vi "Get Groups Channels and Properties from Tags.vi"(6 "error in":errorcluster, 8 "File Tree":string[](array[string]), 9 "tdms file in":refnum<k34>) -> (0 "error out":errorcluster, 1 "channel names out":string[](array[string]), 2 "group names out":string[](array[string]), 3 "tdms file out":refnum<k34>, 4 "property table":string[][](array[string]))   [LabVIEW 2020, in "NI_TDMS File Viewer.lvlib"]
uses:
  <vilib>/Utility/TDMS File Viewer/NI_TDMS File Viewer.lvlib
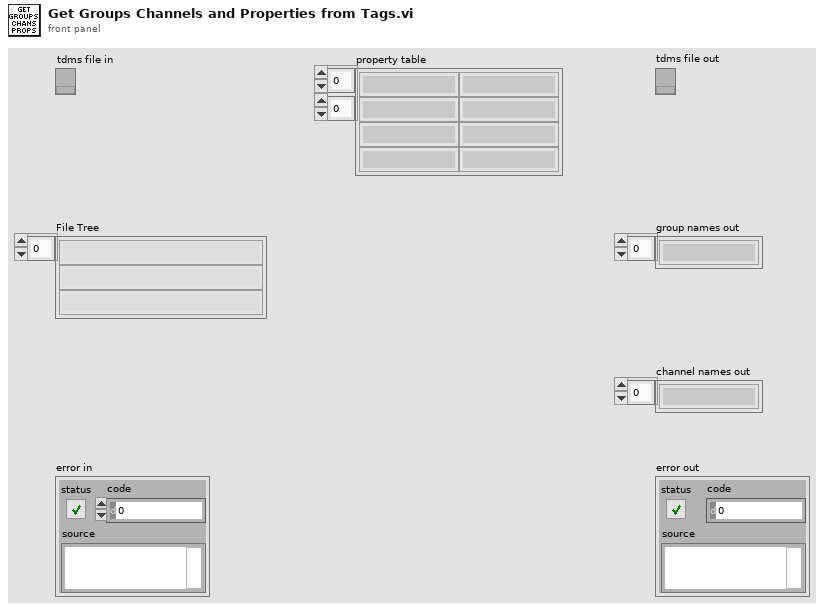
[diagram p1: front panel]
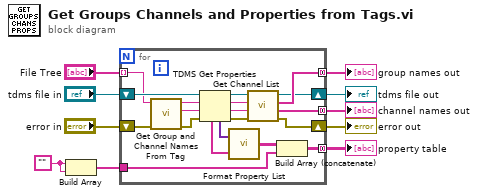
[diagram p0: block diagram]
diagram:
  w7 = "" ("Empty String Constant")
  n1 = Build Array(w7, w7) -> (w8:string[])
  n2 = for {
    tunnel: [w20] -> w1 mode=concatenating
    tunnel: [w19] -> w2 mode=concatenating
    tunnel: "File Tree" -> [w16] mode=indexing
    shift-right: [w28] -> w10
    shift-left: "error in" -> [w26]
    shift-right: [w18] -> w3
    shift-left: "tdms file in" -> [w17]
    tunnel: [w11] -> w6 mode=concatenating
    tunnel: w8 -> [w13]
    n3 = call <vilib>:"Get Group and Channel Names From Tag.vi"("error in"=w26, "tree path"=w16) -> ("error out"=w27:errorcluster, "channel"=w24:string, "group"=w25:string)  [unwired: 3 in]
    n4 = TDMS Get Properties(8:w27, 9:w24, 10:w25, 11:w17) -> (0:w29:errorcluster, 1:w22:string, 2:w21:string, 3:w23:refnum<k34>, 4:w14:variant[], 6:w15:string[])  [unwired: 2 out]
    n5 = call <vilib>:"Format Property List.vi"("property names"=w15, "property values"=w14) -> ("strings"=w12:string[][])
    n6 = call <vilib>:"Get Channel List.vi"("error in"=w29, "channel names"=w22, "group name"=w21, "tdms file"=w23) -> ("error out"=w28:errorcluster, "channel names out"=w20:string[], "group names out"=w19:string[], "tdms file out"=w18:refnum<k34>)
    n7 = Build Array (concatenate)(w12, w13) -> (w11:string[][])
  }
  "property table" <- w6
  "error out" <- w10
  "tdms file out" <- w3
  "group names out" <- w2
  "channel names out" <- w1
